vi "Get Controller Info.vi"(4 "Expose System Hardware Reference":bool caption="Expose System Hardware Reference (F)", 6 "Network Adapters":bool caption="Network Adapters (F)", 8 "error in":errorcluster, 11 "Session in":refnum<k21>="localhost") -> (0 "error out":errorcluster, 2 "Network Device":T1 {"Network Adapter Settings"."IP Address Request Mode" items=["Static"=1, "DHCP/Link Local"=2, "Link-Local Only"=4, "DHCP Only"=8]; "Network Adapter Settings"."Adapter Type" items=["Disabled"=1, "TCP/IP Ethernet"=2, "Deterministic"=4, "EtherCAT"=8, "TCP/IP WLAN Connect"=32, "TCP/IP WLAN Create"=64]; "Network Adapter Settings"."Adapter Mode" items=["Disabled"=1, "TCP/IP Ethernet"=2, "Deterministic"=4, "EtherCAT"=8, "TCP/IP WLAN Connect"=32, "TCP/IP WLAN Create"=64]; "Device Information"."Product ID" format="%.0x"}, 3 "Session out":refnum<k21>="localhost")   [LabVIEW 2015, in "RT Management.lvlib" / "RT Management.lvclass"]
uses:
  RT Management.lvclass
  Distributed Devices/Controls/NetworkDevice.ctl
  Distributed Devices/Controls/DeviceInformation.ctl
  Distributed Devices/Controls/NetworkAdapterSettings.ctl
  <vilib>/nisyscfg/Find Hardware.vi
  <vilib>/nisyscfg/Close (Resources).vi
  <vilib>/nisyscfg/Close (Filter).vi
  <vilib>/nisyscfg/nisyscfg.lvlib
  <resource>/objmgr/niflexriosae.rc
  Distributed Devices/Device.lvclass
  <resource>/objmgr/nisysapi.rc
  RT Management.lvlib
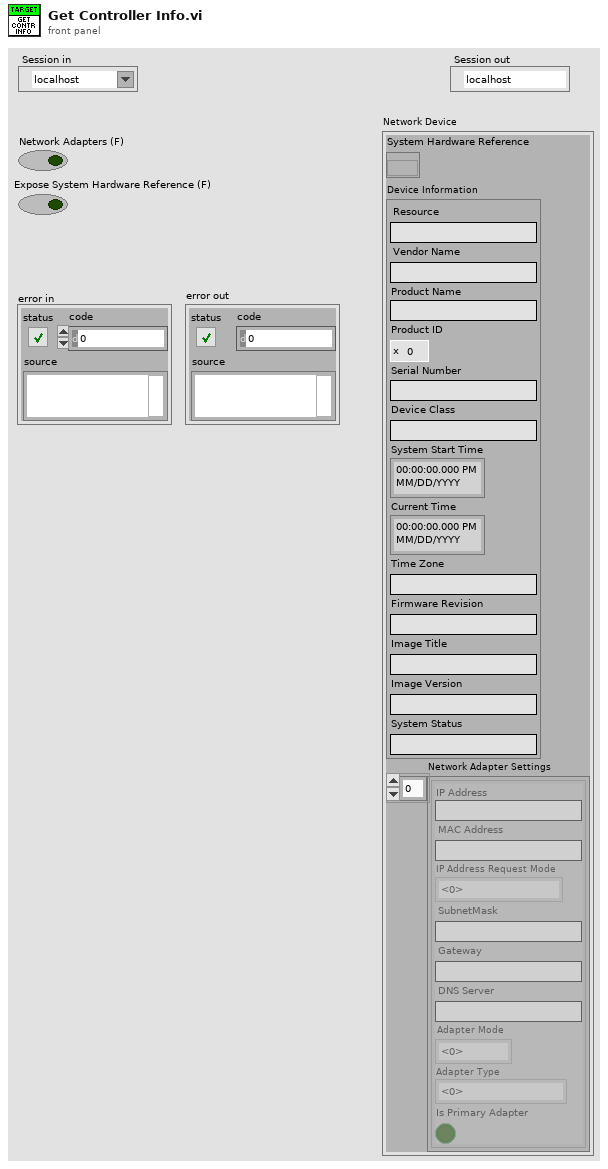
[diagram p1: front panel]
types:
  T1 = typedef "RT Management.lvlib/Device.lvclass/NetworkDevice.ctl" = cluster{"System Hardware Reference":refnum<k20>, "Device Information":T2, "Network Adapter Settings":T3[]}
  T2 = typedef "RT Management.lvlib/Device.lvclass/DeviceInformation.ctl" = cluster{"Resource":string, "Vendor Name":string, "Product Name":string, "Product ID":u32, "Serial Number":string, "Device Class":string, "System Start Time":timestamp, "Current Time":timestamp, "Time Zone":string, "Firmware Revision":string, "Image Title":string, "Image Version":string, "System Status":string}
  T3 = typedef "RT Management.lvlib/Device.lvclass/NetworkAdapterSettings.ctl" = cluster{"IP Address":string, "MAC Address":string, "IP Address Request Mode":u32, "SubnetMask":string, "Gateway":string, "DNS Server":string, "Adapter Mode":u32, "Adapter Type":u32, "Is Primary Adapter":bool}
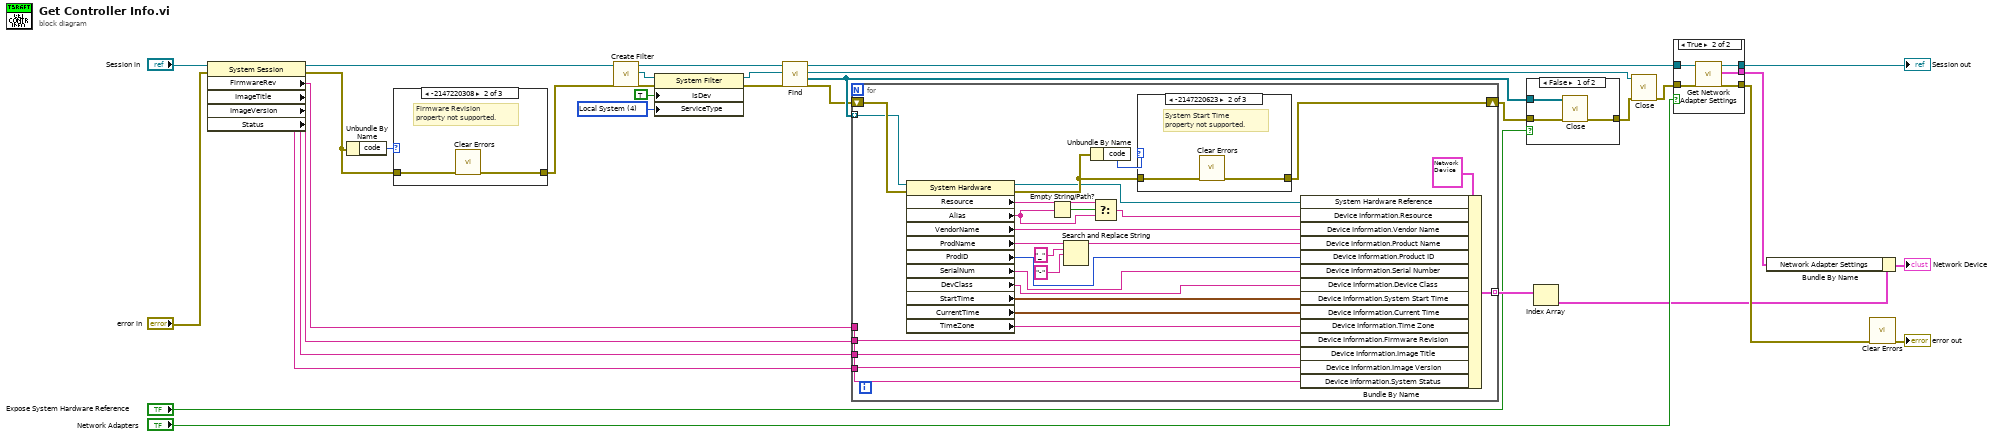
[diagram p0: block diagram]
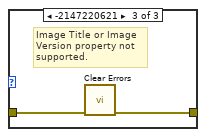
[diagram p3: hidden frame]
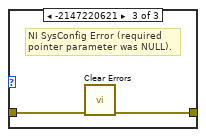
[diagram p6: hidden frame]
diagram:
  w1 = u32 4 items=["NI Network Resource", "NI Real-Time", "NI System Configuration", "NI Web Interface", "Local System", "Local Network Adapter", "Local Time Keeper", "Local Time Reference", "LXI Instrument", "Local FPGA"] ("Service Type")
  n1 = property class="System Session"(reference="Session in", error in="error in") -> (reference out=w5:refnum<k21>, error out=w21:errorcluster, "FirmwareRev"=w14:string, "ImageTitle"=w23:string, "ImageVersion"=w25:string, "Status"=w24:string)
  n2 = Unbundle By Name(w21) -> ("code"=w20:i32)
  n3 = case shown="-2147220308" w20 {
    tunnel: w21 -> [w34 w36 w38]
    tunnel: [w34 w35 w37] -> w6
    frame Default {
    }
    frame -2147220308 {
      # "Firmware Revision\nproperty not supported."
      n4 = call <vilib>:"Clear Errors.vi"("error in (no error)"=w36) -> ("error out"=w35:errorcluster)  [unwired: 5 in, 1 out]
    }
    frame -2147220621 {
      # "Image Title or Image\nVersion property not \nsupported."
      n5 = call <vilib>:"Clear Errors.vi"("error in (no error)"=w38) -> ("error out"=w37:errorcluster)  [unwired: 5 in, 1 out]
    }
  }
  n6 = call <vilib>:"Create Filter.vi"("error in (no error)"=w6, "Session in"=w5) -> ("error out"=w9:errorcluster, "Filter out"=w8:refnum<k20>, "Session out"=w4:refnum<k21>)  [unwired: 7 in]
  n7 = property class="System Filter"(reference=w8, error in=w9, "IsDev"=TRUE ("Is Device"), "ServiceType"=w1) -> (reference out=w3:refnum<k20>, error out=w7:errorcluster)
  n8 = call-poly <vilib>:"Find.vi"("error in (no error)"=w7, "Filter in"=w3, "Session in"=w4) -> ("error out"=w13:errorcluster, "Resources out"=w17:refnum<k20>[], "Filter out"=w18:refnum<k20>, "Session out"=w27:refnum<k21>)  [unwired: 5 in]
  n9 = for {
    tunnel: w25 -> [w65]
    tunnel: w24 -> [w64]
    tunnel: w23 -> [w63]
    tunnel: w17 -> [w40] mode=indexing
    tunnel: [w58] -> w11 mode=indexing
    tunnel: w14 -> [w57]
    shift-right: [w60] -> w16
    shift-left: w13 -> [w56]
    n10 = property class="System Hardware"(reference=w40, error in=w56) -> (reference out=w39:refnum<k20>, error out=w62:errorcluster, "Resource"=w53:string, "Alias"=w52:string, "VendorName"=w49:string, "ProdName"=w47:string, "ProdID"=w44:u32, "SerialNum"=w45:string, "DevClass"=w41:string, "StartTime"=w50:timestamp, "CurrentTime"=w54:timestamp, "TimeZone"=w55:string)
    n11 = Empty String/Path?(string/path=w52) -> (empty?=w51:bool)
    n12 = Search and Replace String(input string=w47, search string="_", replace string="-" ("replace string (\"\")")) -> (result string=w46:string)  [unwired: 5 in, 3 out]
    n13 = Unbundle By Name(w62) -> ("code"=w61:i32)
    n14 = Select(t=w53, s=w51, f=w52) -> (s? t:f=w48:string)
    n15 = case shown="-2147220623" w61 {
      tunnel: w62 -> [w66 w68 w70]
      tunnel: [w66 w67 w69] -> w60
      frame Default {
      }
      frame -2147220623 {
        # "System Start Time\nproperty not supported."
        n16 = call <vilib>:"Clear Errors.vi"("error in (no error)"=w68) -> ("error out"=w67:errorcluster)  [unwired: 5 in, 1 out]
      }
      frame -2147220621 {
        # "NI SysConfig Error (required\npointer parameter was NULL)."
        n17 = call <vilib>:"Clear Errors.vi"("error in (no error)"=w70) -> ("error out"=w69:errorcluster)  [unwired: 5 in, 1 out]
      }
    }
    n18 = Bundle By Name(cluster=T1 {"System Hardware Reference"=refnum, "Device Information"={"Resource"="", "Vendor Name"="", "Product Name"="", "Product ID"=0, "Serial Number"="", "Device Class"="", "System Start Time"=timestamp(0 s since 1904-01-01), "Current Time"=timestamp(0 s since 1904-01-01), "Time Zone"="", "Firmware Revision"="", "Image Title"="", "Image Version"="", "System Status"=""}, "Network Adapter Settings"=[]} ("Network Device"), "System Hardware Reference"=w39, "Device Information.Resource"=w48, "Device Information.Vendor Name"=w49, "Device Information.Product Name"=w46, "Device Information.Product ID"=w44, "Device Information.Serial Number"=w45, "Device Information.Device Class"=w41, "Device Information.System Start Time"=w50, "Device Information.Current Time"=w54, "Device Information.Time Zone"=w55, "Device Information.Firmware Revision"=w57, "Device Information.Image Title"=w63, "Device Information.Image Version"=w65, "Device Information.System Status"=w64) -> (w58:T1)
  }
  n19 = case shown="False" "Expose System Hardware Reference" {
    tunnel: [w73 w74] -> w19
    tunnel: w17 -> [w72 _]
    tunnel: w16 -> [w71 w74]
    frame False {
      n20 = call-poly <vilib>:"Close.vi"("error in (no error)"=w71, "Resources in"=w72) -> ("error out"=w73:errorcluster)  [unwired: 9 in]
    }
    frame True {
    }
  }
  n21 = Index Array(array=w11) -> (element=w12:T1)  [unwired: 1 in]
  n22 = call-poly <vilib>:"Close.vi"("error in (no error)"=w19, "Filter in"=w18) -> ("error out"=w26:errorcluster)  [unwired: 9 in]
  n23 = case shown="True" "Network Adapters" {
    tunnel: w27 -> [w76 w81]
    tunnel: w26 -> [w75 w80]
    tunnel: [_ w79] -> w22
    tunnel: [w76 w78] -> w31
    tunnel: [w75 w77] -> w15
    frame False {
    }
    frame True {
      n24 = call "Get Network Adapter Settings.vi"("error in"=w80, "Refnum in"=w81) -> ("error out"=w77:errorcluster, "Network Adapter Settings"=w79:T3[], "Refnum out"=w78:refnum<k21>)  [unwired: 7 in]
    }
  }
  "Session out" <- w31
  n25 = Bundle By Name(cluster=w12, "Network Adapter Settings"=w22) -> (→"Network Device":T1)
  n26 = call <vilib>:"Clear Errors.vi"("error in (no error)"=w15) -> ("error out"=→"error out":errorcluster)  [unwired: 5 in, 1 out]
